vi "Create Recipe Process.vi"(6 "error in (no error)":errorcluster, 7 "Recipe Controller.lvclass":refnum<class "Recipe Controller.lvclass">, 8 "2-Axis Stage Async API.lvclass":refnum<class "2-Axis Stage Async API.lvclass">, 9 "DAQ API.lvclass":refnum<class "DAQ API.lvclass">, 10 "Camera Controller":refnum<class "Camera Controller.lvclass">, 11 "Laser API.lvclass":refnum<class "Laser API.lvclass">) -> (0 "error out":errorcluster, 3 "Recipe Controller.lvclass":refnum<class "Recipe Controller.lvclass">)   [LabVIEW 2022 SP3, in "Recipe Process.lvlib" / "Recipe Process.lvclass"]
uses:
  Recipe Process.lvclass
  Recipe Controller/Recipe Controller.lvclass
  Camera/Camera Controller/Camera Controller.lvclass
  Laser/Laser Controller api/Laser API.lvclass
  IO Monitor/DAQ API/DAQ API.lvclass
  XY Stage/Interfaces/2-Axis Stage API/2-Axis Stage Async API.lvclass
  C:/Program Files/National Instruments/LabVIEW 2022/vi.lib/ActorFramework/Actor/Actor.lvclass
  Recipe Process.lvclass/Recipe Process.ctl
  <vilib>/ActorFramework/Actor/Actor.lvclass
  XY Stage/Process Actor/Process Framework/Process State Data/Process State Data.lvclass
  XY Stage/Process Actor/Process Framework/Interlock Q Class/Interlock Q Class.lvclass
  Recipe State Data/Recipe State Data.lvclass
  C:/Program Files/National Instruments/LabVIEW 2022/vi.lib/MGI/Monitored Actor/Monitored Actor/Monitored Actor/Monitored Actor.lvclass
  C:/XY Stage/Process Actor Project/Recipe Process/Recipe Process/Recipe Process.lvclass
  C:/XY Stage/Process Actor Project/Recipe/Recipe.lvclass
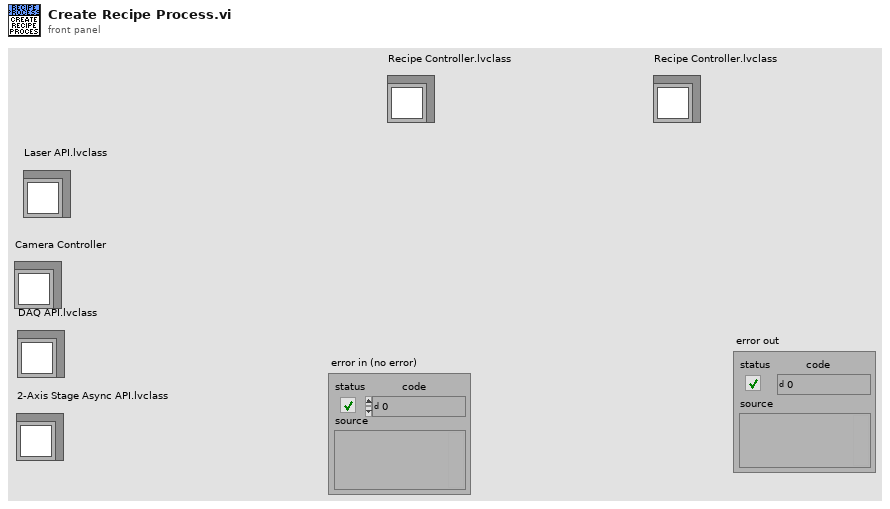
[diagram p1: front panel]
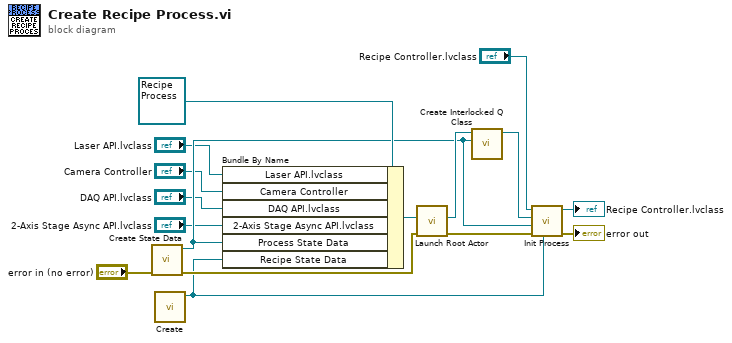
[diagram p0: block diagram]
diagram:
  n1 = call "Create State Data.vi"("error in (no error)"="error in (no error)") -> ("error out"=w6:errorcluster, "Process State Data out"=w8:refnum<data-value>)  [unwired: 9 in]
  n2 = call "Create.vi"() -> ("Recipe State Data"=w1:refnum<data-value>)  [unwired: 11 in]
  n3 = Bundle By Name(cluster=refnum<class "Recipe Process.lvclass"> refnum ("Recipe Process.lvlib:Recipe Process.lvclass"), "Laser API.lvclass"="Laser API.lvclass", "Camera Controller"="Camera Controller", "DAQ API.lvclass"="DAQ API.lvclass", "2-Axis Stage Async API.lvclass"="2-Axis Stage Async API.lvclass", "Process State Data"=w8, "Recipe State Data"=w1) -> (w15:refnum<class "Recipe Process.lvclass">)
  n4 = call <vilib>:"Launch Root Actor.vi"("error in (no error)"=w6, "Actor"=w15) -> ("error out"=w7:errorcluster, "Actor's Enqueuer"=w13:refnum<class "Message Enqueuer.lvclass">)  [unwired: 8 in]
  n5 = call "Create Interlocked Q Class.vi"("Process State Data"=w8, "Process Q"=w13) -> ("Interlock Q Class out"=w12:refnum<class "Interlock Q Class.lvclass">)  [unwired: 9 in]
  n6 = call "Init Process.vi"("Recipe State Data"=w1, "error in (no error)"=w7, "Process State Data"=w8, "Interlock Q Class"=w12, "Recipe Controller in"="Recipe Controller.lvclass") -> ("error out"=→"error out":errorcluster, "Recipe Controller out"=→"Recipe Controller.lvclass":refnum<class "Recipe Controller.lvclass">)  [unwired: 5 in]
